vi "Analyze Hierarchy for Reentrancy_Pretest.vi"(6 "error in (no error)":errorcluster, 7 "Flattenned Parameters in":string[](array[string]), 10 "Require Preallocated Reentrancy":bool=TRUE, 11 "Test Name":string) -> (0 "error out":errorcluster, 1 "Flattenned Parameters out":string[](array[string]), 2 "Array":T1[](array[typedef])=[{"VI Name"="MC_CommandStatement_break.vi", "Path"=path "C:/Program Files/National Instruments/LabVIEW 2009/vi.lib/imath/engines/lvmath2/RunTimeEngine/CommandStatement/MC_CommandStatement_break.vi", "Reentrant"=FALSE, "Execution:Reentrancy Type"=enum."Share clones between instances", "Execution:Preferred Exec System"=enum."invalid execution system", "Exec.Priority"=enum."invalid priority"}, {"VI Name"="NIMS_NodeEndStatement_Output.vi", "Path"=path "C:/Program Files/National Instruments/LabVIEW 2009/vi.lib/imath/engines/lvmath2/RunTimeEngine/NodeEndStatement/NIMS_NodeEndStatement_Output.vi", "Reentrant"=TRUE, "Execution:Reentrancy Type"=enum."Share clones between instances", "Execution:Preferred Exec System"=enum."invalid execution system", "Exec.Priority"=enum."invalid priority"}, {"VI Name"="NIMS_NodeEndStatement_Output_B70DDD75627E4997AAE11E9955EDAA25_000.vi", "Path"=path "C:/Documents and Settings/rgosalia/My Documents/LabVIEW Data/InstCache/9.0/0/NIMS_NodeEndStatement_Output_B70DDD75627E4997AAE11E9955EDAA25.lvgen/NIMS_NodeEndStatement_Output_B70DDD75627E4997AAE11E9955EDAA25_000.vi", "Reentrant"=TRUE, "Execution:Reentrancy Type"=enum."Share clones between instances", "Execution:Preferred Exec System"=enum."invalid execution system", "Exec.Priority"=enum."invalid priority"}, {"VI Name"="NIMS_Finalize Error.vi", "Path"=path "C:/Program Files/National Instruments/LabVIEW 2009/vi.lib/imath/engines/lvmath2/RunTimeEngine/ErrorHandling/NIMS_Finalize Error.vi", "Reentrant"=FALSE, "Execution:Reentrancy Type"=enum."Share clones between instances", "Execution:Preferred Exec System"=enum."invalid execution system", "Exec.Priority"=enum."invalid priority"}, {"VI Name"="Untranslate Error.vi", "Path"=path "C:/Program Files/National Instruments/LabVIEW 2009/vi.lib/imath/engines/lvmath/Functions/Error Handling/Untranslate Error.vi", "Reentrant"=FALSE, "Execution:Reentrancy Type"=enum."Preallocate clone for each instance", "Execution:Preferred Exec System"=enum."invalid execution system", "Exec.Priority"=enum."invalid priority"}, {"VI Name"="MC_GlobalManager.vi", "Path"=path "C:/Program Files/National Instruments/LabVIEW 2009/vi.lib/imath/engines/lvmath2/RunTimeEngine/Managers/GlobalManager/MC_GlobalManager.vi", "Reentrant"=FALSE, "Execution:Reentrancy Type"=enum."Preallocate clone for each instance", "Execution:Preferred Exec System"=enum."invalid execution system", "Exec.Priority"=enum."invalid priority"}, {"VI Name"="NIMS_KS_Error Code Database.vi", "Path"=path "C:/Program Files/National Instruments/LabVIEW 2009/vi.lib/imath/engines/lvmath2/MathScriptCompiler/Dependencies/error.llb/NIMS_KS_Error Code Database.vi", "Reentrant"=FALSE, "Execution:Reentrancy Type"=enum."Preallocate clone for each instance", "Execution:Preferred Exec System"=enum."invalid execution system", "Exec.Priority"=enum."invalid priority"}, {"VI Name"="MC_Register_VI_In_Memory.vi", "Path"=path "C:/Program Files/National Instruments/LabVIEW 2009/vi.lib/imath/engines/lvmath2/RunTimeEngine/Managers/GlobalRegistration/MC_Register_VI_In_Memory.vi", "Reentrant"=FALSE, "Execution:Reentrancy Type"=enum."Preallocate clone for each instance", "Execution:Preferred Exec System"=enum."invalid execution system", "Exec.Priority"=enum."invalid priority"}, {"VI Name"="MC_Get_Notification_Event.vi", "Path"=path "C:/Program Files/National Instruments/LabVIEW 2009/vi.lib/imath/engines/lvmath2/RunTimeEngine/Managers/GlobalRegistration/MC_Get_Notification_Event.vi", "Reentrant"=FALSE, "Execution:Reentrancy Type"=enum."Preallocate clone for each instance", "Execution:Preferred Exec System"=enum."invalid execution system", "Exec.Priority"=enum."invalid priority"}, {"VI Name"="MC_Registered_VIs_Global.vi", "Path"=path "C:/Program Files/National Instruments/LabVIEW 2009/vi.lib/imath/engines/lvmath2/RunTimeEngine/Managers/GlobalRegistration/MC_Registered_VIs_Global.vi", "Reentrant"=FALSE, "Execution:Reentrancy Type"=enum."Preallocate clone for each instance", "Execution:Preferred Exec System"=enum."invalid execution system", "Exec.Priority"=enum."invalid priority"}, {"VI Name"="MC_Version.vi", "Path"=path "C:/Program Files/National Instruments/LabVIEW 2009/vi.lib/imath/engines/lvmath2/RunTimeEngine/Parser/MC_Version.vi", "Reentrant"=FALSE, "Execution:Reentrancy Type"=enum."Share clones between instances", "Execution:Preferred Exec System"=enum."invalid execution system", "Exec.Priority"=enum."invalid priority"}], 3 "Worked?":bool, 4 "Reentrancy OK?":bool, 5 "Preferred Exec System OK?":bool)   [LabVIEW 2009]
uses:
  VI Reentrancy Setting.ctl
  CommonSubVIs/Framework/Flattened_Array/Test Parameter Enum.ctl
  CommonSubVIs/Framework/Flattened_Array/Set Parameter Value by Name (Variant).vi
  CommonSubVIs/Framework/Flattened_Array/Set Parameter Value by Name (Bool).vi
  CommonSubVIs/Framework/Flattened_Array/Get Parameter Value by Name (Bool).vi
  CommonSubVIs/Framework/Flattened_Array/Get Parameter Value by Name (String).vi
panel:
  in  "Tab Control":enum32{"Setup", "Results", "Framework Stuff"}(tab)
  in  "Require 'Same as Caller'\nExec System Setting":bool=TRUE
  out "Exec System Setting Problems":string[](array[string])
  out "Reentrancy Problems":string[](array[string])
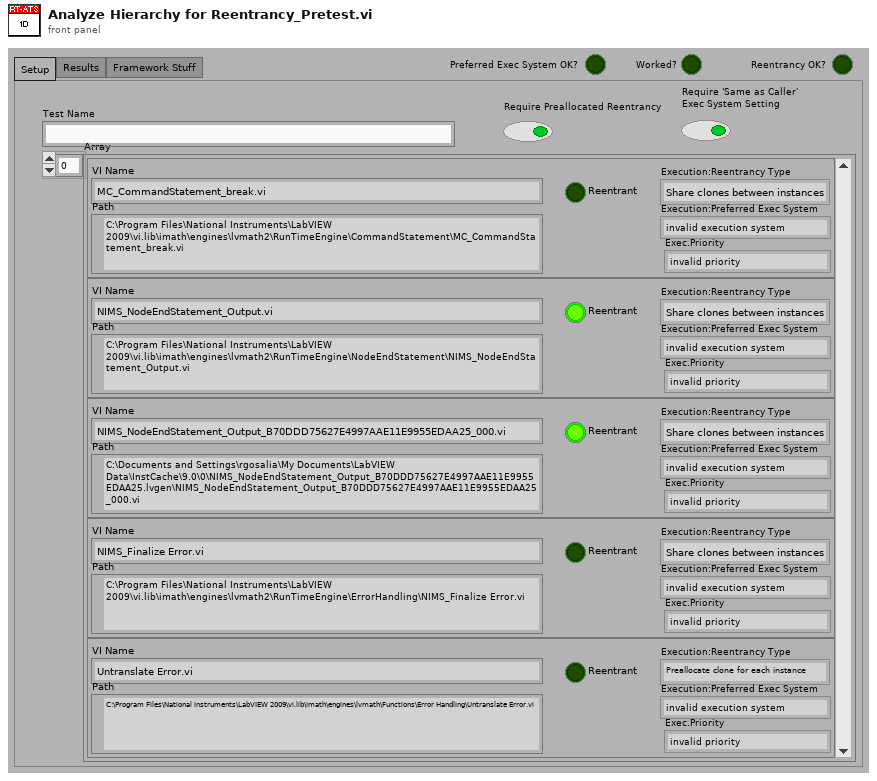
[diagram p1: front panel]
types:
  T1 = typedef "VI Reentrancy Setting.ctl" = cluster{"VI Name":string, "Path":path, "Reentrant":bool, "Execution:Reentrancy Type":enum16{"Share clones between instances", "Preallocate clone for each instance"}, "Execution:Preferred Exec System":enum32{"invalid execution system", "user interface", "standard", "instrument i/o", "data acquisition", "other 1", "other 2", "same as caller"}, "Exec.Priority":enum32{"invalid priority", "background priority", "normal priority", "above normal priority", "high priority", "time critical priority", "subroutine"}}
  T2 = typedef "Test Parameter Enum.ctl" = enum16{"Main Test Target IP", "Main Test Target Name", "Main Test Target Alias", "Main Host IP", "Default Target Alias", "Default Target Host Name", "Dafault Target IP Address", "Dafault Target LV Date", "Available Targets", "Target Alias by Index", "Target IP by Alias", "Current Iteration", "Total Iterations", "Test Project Name", "Current Test Result", "Current Test Name", "Current Test Logical Path", "Test Folder", "Configuration Name", "Configuration Index", "Total Configurations", "Performance Values", "Result Paragraphs", "Connector Pane", "Avoid?", "Avoid Reason", "Case Name", "Case #", "Total Cases", "Case Data"}
  T3 = enum32{"invalid priority", "background priority", "normal priority", "above normal priority", "high priority", "time critical priority", "subroutine"}
  T4 = enum32{"invalid execution system", "user interface", "standard", "instrument i/o", "data acquisition", "other 1", "other 2", "same as caller"}
  T5 = enum16{"Share clones between instances", "Preallocate clone for each instance"}
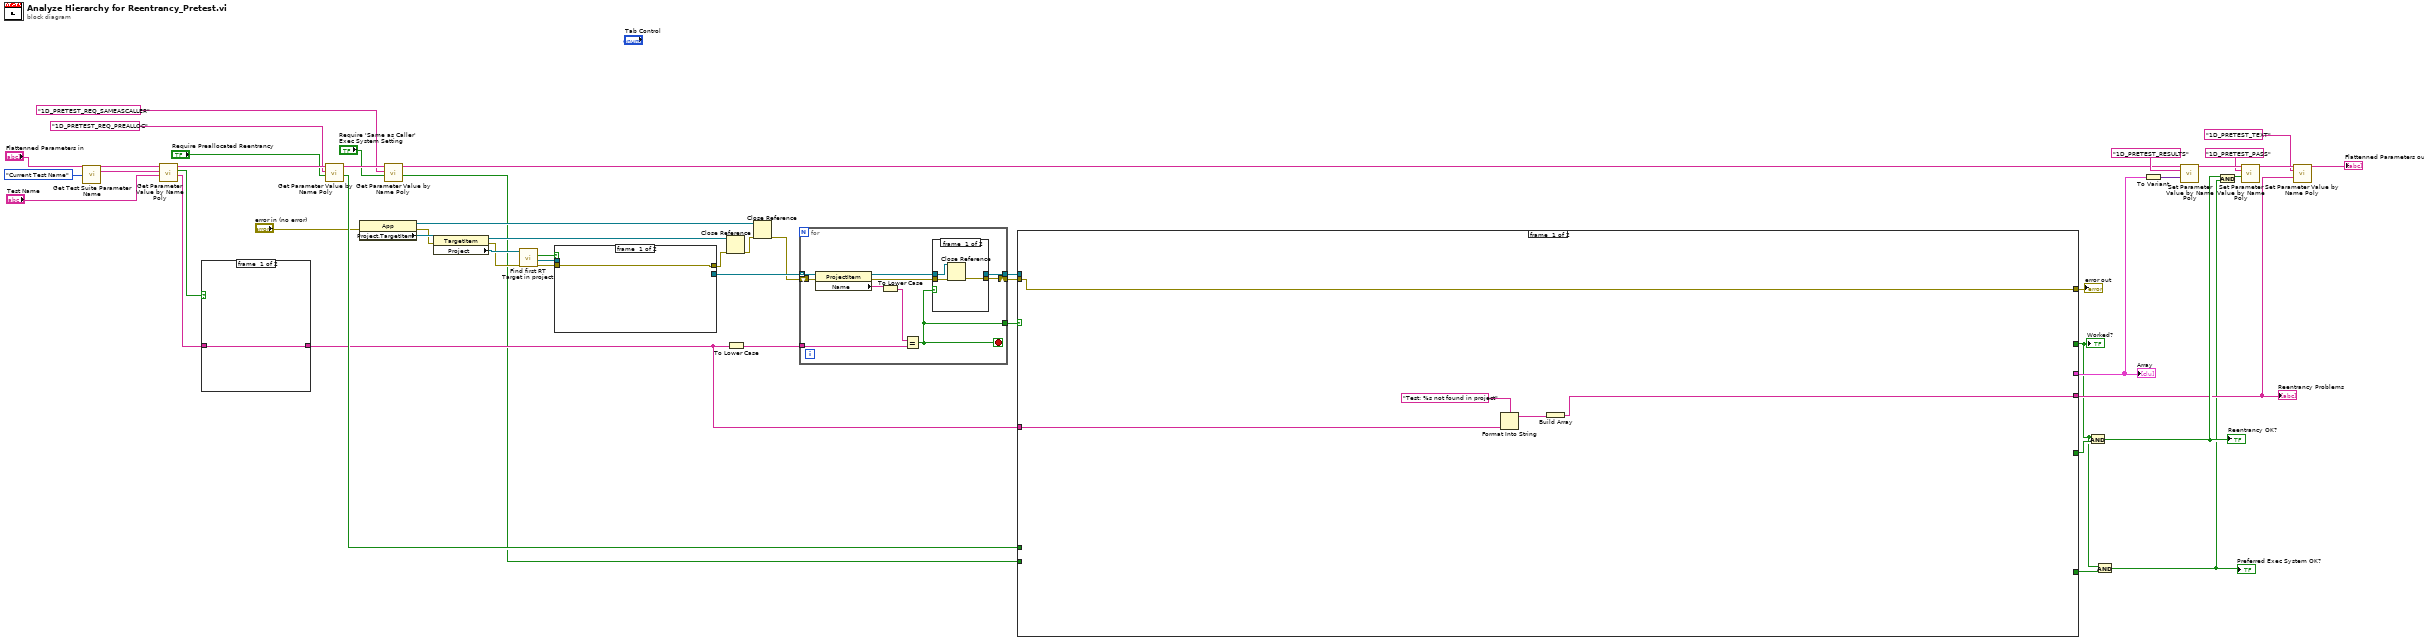
[diagram p0: block diagram]
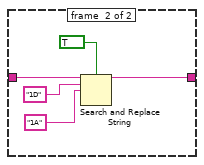
[diagram p2: hidden frame]
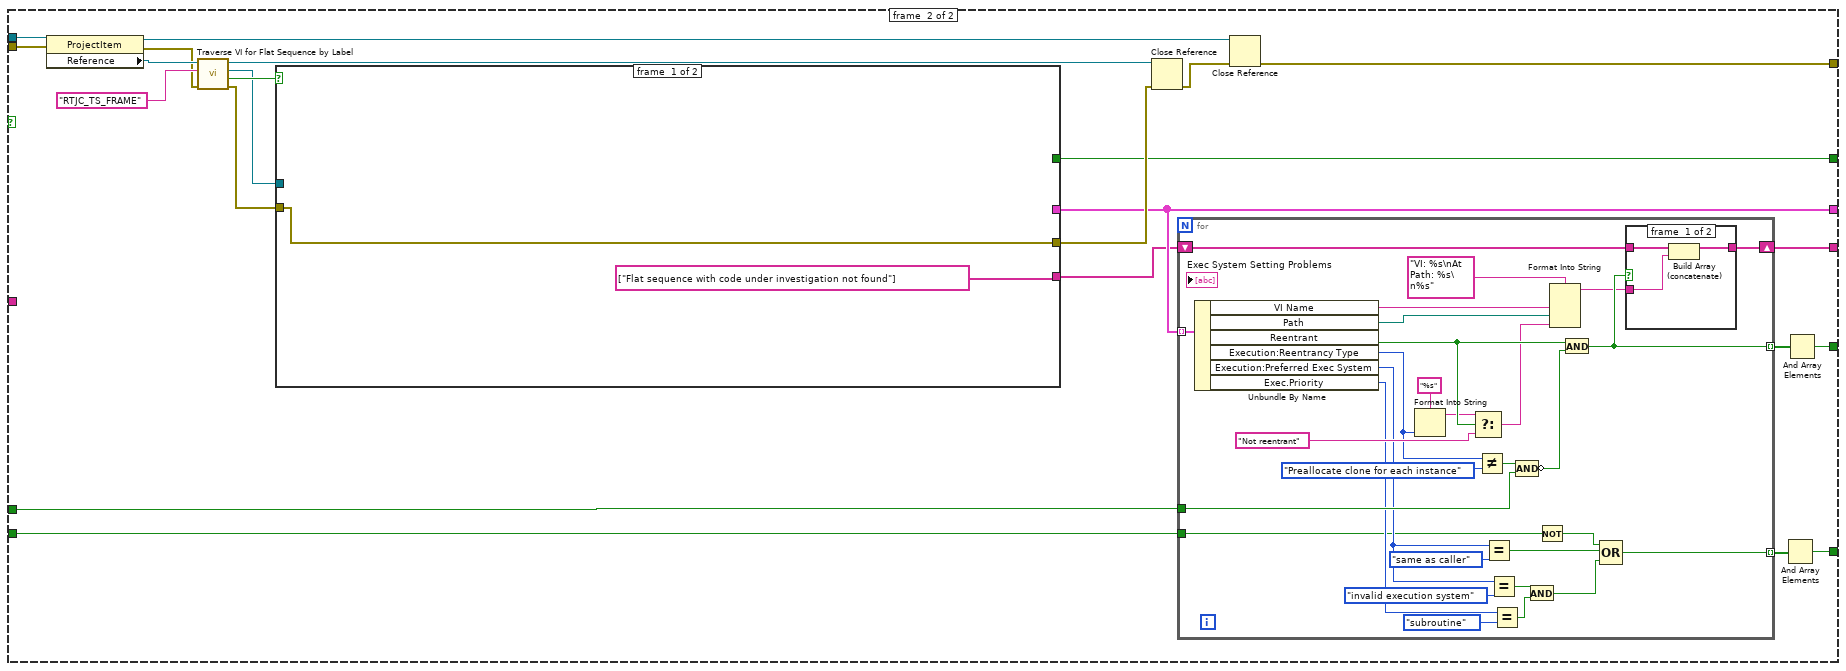
[diagram p3: hidden frame]
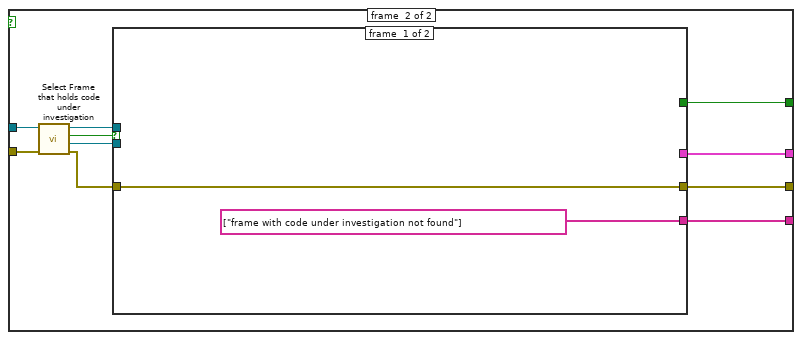
[diagram p5: hidden frame]
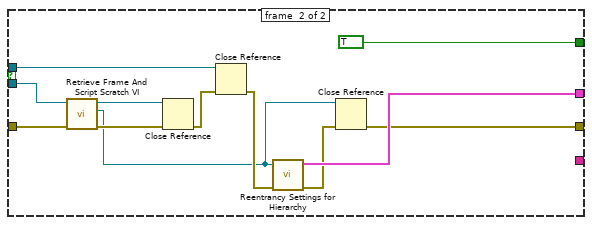
[diagram p6: hidden frame]
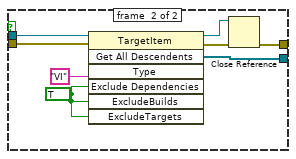
[diagram p8: hidden frame]
diagram:
  n1 = call "Get Test Suite Parameter Name.vi"("Test Suite Parameter"=Test_Parameter_Enum."Current Test Name") -> ("Parameter Name"=w49:string)  [unwired: 13 in, 1 out]
  n2 = call-poly "Get Parameter Value by Name Poly.vi"("Default Value"="Test Name", "Parameter"=w49, "Parameter Array in"="Flattenned Parameters in") -> ("Value"=w12:string, "Found?"=w13:bool, "Parameter Array Out"=w20:string[])  [unwired: 5 in]
  n3 = case shown="False" w13 {
    tunnel: w12 -> [w51 w55]
    tunnel: [w51 w53] -> w11
    frame #0 {
    }
    frame #1 {
      n4 = Search and Replace String(case sensitive?=TRUE ("ignore case? (F)"), input string=w55, search string="1D", replace string="1A" ("search string")) -> (result string=w53:string)  [unwired: 4 in, 3 out]
    }
  }
  n5 = call-poly "Get Parameter Value by Name Poly.vi"("Default Value"="Require Preallocated Reentrancy", "Parameter"="1D_PRETEST_REQ_PREALLOC" ("Parameter Name"), "Parameter Array in"=w20) -> ("Value"=w17:bool, "Parameter Array Out"=w9:string[])  [unwired: 5 in, 1 out]
  n6 = property class="App"(error in="error in (no error)") -> (reference out=w36:refnum<vi>, error out=w41:errorcluster, "Project.TargetItem"=w46:refnum<vi>)  [unwired: 1 in]
  n7 = call-poly "Get Parameter Value by Name Poly.vi"("Default Value"="Require 'Same as Caller'\nExec System Setting", "Parameter"="1D_PRETEST_REQ_SAMEASCALLER" ("Parameter Name"), "Parameter Array in"=w9) -> ("Value"=w5:bool, "Parameter Array Out"=w8:string[])  [unwired: 5 in, 1 out]
  n8 = property class="TargetItem"(reference=w46, error in=w41) -> (reference out=w39:refnum<vi>, error out=w42:errorcluster, "Project"=w45:refnum<vi>)
  n9 = call "Find first RT Target in project.vi"("error in"=w42, "Project Refnum"=w45) -> ("error out"=w40:errorcluster, "Target"=w44:refnum<vi>, "Found?"=w43:bool)  [unwired: 6 in, 1 out]
  n10 = case shown="True" w43 {
    tunnel: w44 -> [_ w65]
    tunnel: [_ w62] -> w35
    tunnel: [w57 w58] -> w38
    tunnel: w40 -> [w57 w61]
    frame #0 {
    }
    frame #1 {
      w64 = TRUE ("ExcludeDependencies")
      n11 = invoke class="TargetItem" method="Get All Descendents"(reference=w65, error in=w61, "Type"="VI", "Exclude Dependencies"=w64, "ExcludeBuilds"=w64, "ExcludeTargets"=w64) -> (reference out=w59:refnum<vi>, error out=w60:errorcluster, "All Descendents"=w62:refnum<vi>[])  [unwired: 1 in, 4 out]
      n12 = Close Reference(reference=w59, error in (no error)=w60) -> (error out=w58:errorcluster)
    }
  }
  n13 = Close Reference(reference=w39, error in (no error)=w38) -> (error out=w37:errorcluster)
  n14 = To Lower Case(string=w11) -> (all lower case string=w33:string)
  n15 = Close Reference(reference=w36, error in (no error)=w37) -> (error out=w34:errorcluster)
  n16 = for {
    tunnel: w35 -> [w75] mode=indexing
    shift-right: [w67] -> w30
    shift-left: w34 -> [w74]
    tunnel: w33 -> [w72]
    tunnel: [w70] -> w32
    tunnel: [w66] -> w31
    stop <- w70 stop-if-true
    n17 = property class="ProjectItem"(reference=w75, error in=w74) -> (reference out=w68:refnum<vi>, error out=w69:errorcluster, "Name"=w73:string)
    n18 = To Lower Case(string=w73) -> (all lower case string=w71:string)
    n19 = Equal?(x=w71, y=w72) -> (x = y?=w70:bool)
    n20 = case shown="True" w70 {
      tunnel: w69 -> [w78 w80]
      tunnel: w68 -> [w77 w79]
      tunnel: [w76 w80] -> w67
      tunnel: [_ w79] -> w66
      frame #0 {
        n21 = Close Reference(reference=w77, error in (no error)=w78) -> (error out=w76:errorcluster)
      }
      frame #1 {
      }
    }
  }
  n22 = case shown="True" w32 {
    tunnel: w31 -> [_ w102]
    tunnel: w30 -> [w85 w101]
    tunnel: [w85 w98] -> w27
    tunnel: [_ w97] -> w28
    tunnel: [_ w95] -> w24
    tunnel: [_ w92] -> w3
    tunnel: w17 -> [_ w91]
    tunnel: [w81 w90] -> w16
    tunnel: w11 -> [w84 _]
    tunnel: w5 -> [_ w88]
    tunnel: [_ w86] -> w4
    frame #0 {
      n23 = Format Into String(format string="Test: %s not found in project", w84) -> (resulting string=w82:string)  [unwired: 2 in, 1 out]
      n24 = Build Array(w82) -> (w81:string[])
    }
    frame #1 {
      n25 = property class="ProjectItem"(reference=w102, error in=w101) -> (reference out=w99:refnum<vi>, error out=w103:errorcluster, "Reference"=w108:refnum<vi>)
      n26 = call "Traverse VI for Flat Sequence by Label.vi"("error in"=w103, "Label"="RTJC_TS_FRAME" ("y"), "VI Reference"=w108) -> ("error out"=w93:errorcluster, "Found?"=w106:bool, "FlatSeq Refnum"=w94:refnum<vi>, "VI Reference"=w105:refnum<vi>)  [unwired: 5 in]
      n27 = case shown="True" w106 {
        tunnel: w94 -> [_ w152]
        tunnel: [w144 w154] -> w104
        tunnel: [_ w153] -> w97
        tunnel: w93 -> [w144 w151]
        tunnel: [_ w146] -> w92
        tunnel: [string[] ["Flat sequence with code under investigation not found"] w145] -> w89
        frame #0 {
        }
        frame #1 {
          n28 = call "Select Frame that holds code under investigation.vi"("error in"=w151, "FlatSeq Refnum"=w152) -> ("error out"=w149:errorcluster, "Frame"=w150:refnum<vi>, "OK?"=w147:bool, "FlatSeq Refnum"=w148:refnum<vi>)  [unwired: 6 in]
          n29 = case shown="False" w147 {
            tunnel: [w156 w158] -> w154
            tunnel: [_ w160] -> w153
            tunnel: w150 -> [_ w162]
            tunnel: w149 -> [w156 w165]
            tunnel: w148 -> [_ w164]
            tunnel: [_ TRUE] -> w146
            tunnel: [string[] ["frame with code under investigation not found"] _] -> w145
            frame #0 {
            }
            frame #1 {
              n30 = call "Retrieve Frame And Script Scratch VI.vi"("error in"=w165, "FlatSeqFrame Refnum"=w162) -> ("error out"=w168:errorcluster, "scratch VI"=w157:refnum<vi>, "FlatSeqFrame Refnum (out)"=w167:refnum<vi>)  [unwired: 7 in]
              n31 = Close Reference(reference=w167, error in (no error)=w168) -> (error out=w166:errorcluster)
              n32 = Close Reference(reference=w164, error in (no error)=w166) -> (error out=w161:errorcluster)
              n33 = call "Reentrancy Settings for Hierarchy.vi"("error in"=w161, "Scratch VI"=w157) -> ("error out"=w159:errorcluster, "Reentrancy Settings for VI Hierarchy"=w160:T1[])  [unwired: 8 in]
              n34 = Close Reference(reference=w157, error in (no error)=w159) -> (error out=w158:errorcluster)
            }
          }
        }
      }
      n35 = Close Reference(reference=w105, error in (no error)=w104) -> (error out=w100:errorcluster)
      n36 = for {
        tunnel: w97 -> [w138] mode=indexing
        tunnel: [w125] -> w96 mode=indexing
        tunnel: w91 -> [w136]
        shift-right: [w124] -> w90
        shift-left: w89 -> [w123]
        tunnel: w88 -> [w111]
        tunnel: [w110] -> w87 mode=indexing
        n37 = Unbundle By Name(w138) -> ("VI Name"=w131:string, "Path"=w134:path, "Reentrant"=w132:bool, "Execution:Reentrancy Type"=w120:T5, "Execution:Preferred Exec System"=w119:T4, "Exec.Priority"=w117:T3)
        n38 = Format Into String(format string="%s", w120) -> (resulting string=w130:string)  [unwired: 2 in, 1 out]
        n39 = Select(t=w130, s=w132, f="Not reentrant") -> (s? t:f=w128:string)
        n40 = Not Equal?(x=w120, y=T5."Preallocate clone for each instance" ("Required Reentrancy")) -> (x != y?=w137:bool)
        n41 = Equal?(x=w119, y=T4."same as caller") -> (x = y?=w113:bool)
        n42 = Equal?(x=w119, y=T4."invalid execution system") -> (x = y?=w115:bool)
        n43 = Equal?(x=w117, y=T3."subroutine") -> (x = y?=w114:bool)
        n44 = Compound Arithmetic op=AND(w137, w136) -> (invert w135:bool)
        n45 = And(x=w115, y=w114) -> (x .and. y?=w112:bool)
        n46 = Not(x=w111) -> (.not. x?=w109:bool)
        n47 = Format Into String(format string="VI: %s\nAt Path: %s\n%s", w131, w134, w128) -> (resulting string=w122:string)  [unwired: 2 in, 1 out]
        n48 = And(x=w132, y=w135) -> (x .and. y?=w125:bool)
        n49 = Compound Arithmetic op=OR(w109, w113, w112) -> (w110:bool)
        n50 = case shown="False" w125 {
          tunnel: [w141 w142] -> w124
          tunnel: w123 -> [w140 w142]
          tunnel: w122 -> [w139 _]
          frame #0 {
            n51 = Build Array (concatenate)(w140, w139) -> (w141:string[])
          }
          frame #1 {
          }
        }
      }
      n52 = Close Reference(reference=w99, error in (no error)=w100) -> (error out=w98:errorcluster)
      n53 = And Array Elements(Boolean array=w87) -> (logical AND=w86:bool)
      n54 = And Array Elements(Boolean array=w96) -> (logical AND=w95:bool)
    }
  }
  "Worked?" <- w3
  "error out" <- w27
  "Array" <- w28
  "Reentrancy Problems" <- w16
  n55 = And(x=w3, y=w24) -> (x .and. y?=w23:bool)
  "Reentrancy OK?" <- w23
  n56 = And(x=w3, y=w4) -> (x .and. y?=w1:bool)
  "Preferred Exec System OK?" <- w1
  n57 = To Variant(anything=w28) -> (Variant=w29:variant)
  n58 = call-poly "Set Parameter Value by Name Poly.vi"("Parameter Array"=w8, "Parameter Name"="1D_PRETEST_RESULTS", "Double"=w29) -> ("Parameter Array Out"=w25:string[])  [unwired: 9 in, 3 out]
  n59 = And(x=w23, y=w1) -> (x .and. y?=w2:bool)
  n60 = call-poly "Set Parameter Value by Name Poly.vi"("Parameter Array"=w25, "Parameter Name"="1D_PRETEST_PASS", "Bool"=w2) -> ("Parameter Array Out"=w21:string[])  [unwired: 9 in, 3 out]
  n61 = call-poly "Set Parameter Value by Name Poly.vi"("Parameter Array"=w21, "Parameter Name"="1D_PRETEST_TEXT", "Double"=w16) -> ("Parameter Array Out"=→"Flattenned Parameters out":string[])  [unwired: 9 in, 3 out]
